vi "ARN Test Konfig.vi"() -> ()   [LabVIEW 2020, in "EPA 1065.lvlib" / "ARN Test 1065-305.lvlib"]
uses:
  ARN Test 1065-305.lvlib
  Allgemein/allgemeine Sub-VIs.lvlib
  Aktion FGV ARN Daten.ctl
  Seiten/FT-IR/FT-IR.lvlib
  Seiten/FT-IR/FGV FT-IR Gasliste Aktionen.ctl
  Messdaten/Aktionen FGV Messdaten.ctl
  Messdaten/Messdaten.lvlib
  Aktion FGV ARN Test.ctl
  Seiten/Grafik/Grafik.lvlib
  Aktion FGV ARN Protokoll.ctl
  Funktionstasten/Funktionstasten.lvlib
  Funktionstasten/Funktionstasten-Aktion.ctl
  Funktionstasten/Zustaende.ctl
  Seiten/Gaszuordnung AO/Gaszuordnung AO.lvlib
  Seiten/Gaszuordnung AO/FGV Gaszuordnung Grenzen&Einheit Aktion.ctl
  Aktion FGV ARN-Protokolleinstellungen.ctl
  Aktion FGV Protokoll.ctl
  ARN Info.ctl
  Visualisierungs Elemente/String - Ausgabefeld.ctl
panel:
  out "E_Rauschen:":sgl format="%#.4g"
  out "E_Wiederholgenauigkeit:":sgl format="%#.4g"
  out "E_Genauigkeit:":sgl format="%#.4g"
  out "Rauschen:":sgl caption="Noise:" format="%#.4g"
  out "Wiederholbarkeit:":sgl format="%#.4g"
  out "Genauigkeit:":sgl caption="Accuracy:" format="%#.4g"
  out "Komponente":T1
  out "Mwert":sgl format="%.3f"
  out "PMwert":sgl format="%.3f"
  out "Wert 1":sgl caption="Konzentration" format="%#.3f"
  out "Graph1":waveform(dbl)(graph)
  in  "Abbrechen":bool caption="Cancel"
  out "Status":string
  out "Tabelle":string[][](table)
  in  "SNR Info":T2 {"Konzentration:" format="%#_5g"; "Gas Aufschaltzeit:" format="%#_5g"}
  in  "Textname:":string
  in  "Pfad:":path=path "D:/IAG_Data/Log" caption="Path:"
  in  "Test Start":bool
  in  "Speichern":bool caption="Save"
  # "ARN Test"
  # "Settings"
  # "Graphic"
  # "Limits:"
  # "Results:"
  # "Accuracy:"
  # "Repeatability:"
  # "Noise:"
  # "±"
  # "x"
  # "Protocol settings"
  # "ARN Test"
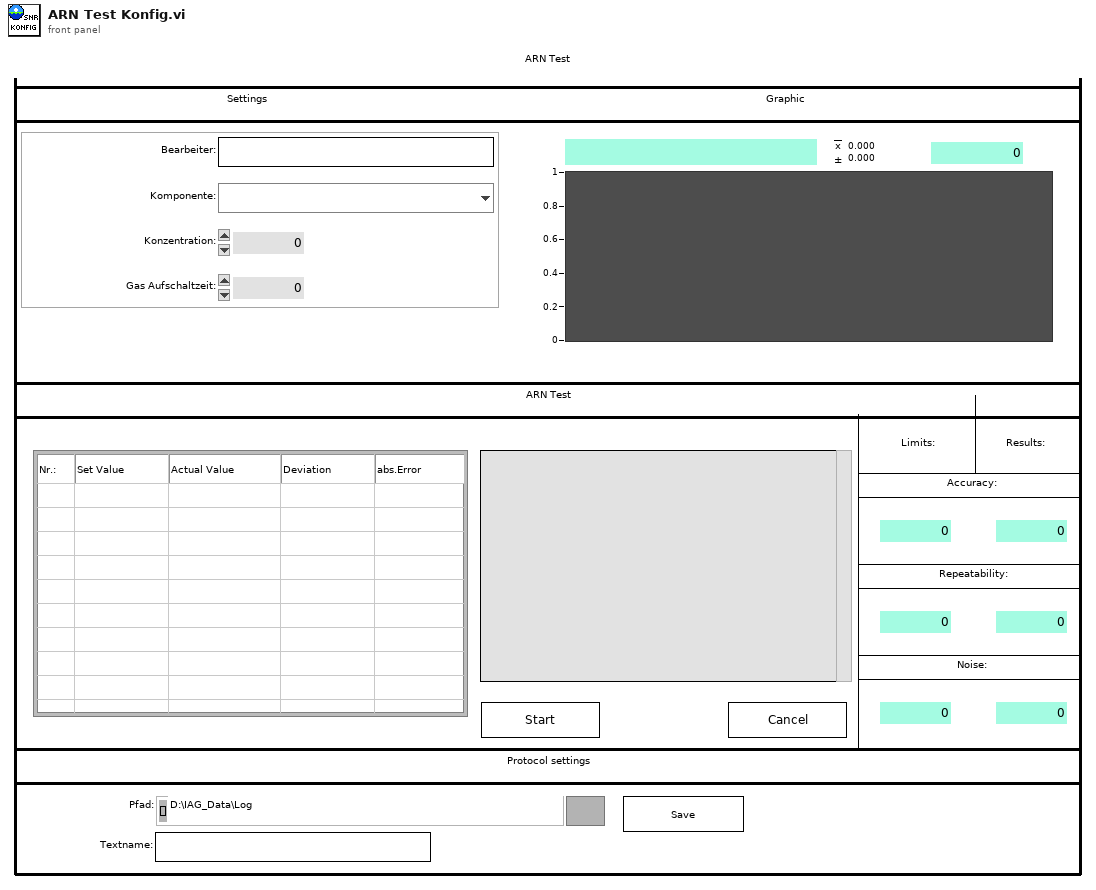
[diagram p1: front panel]
types:
  T1 = typedef "String - Ausgabefeld.ctl" = string
  T2 = typedef "EPA 1065.lvlib/ARN Test 1065-305.lvlib/ARN Info.ctl" = cluster{"Bearbeiter:":string, "Komponente:":u16, "Konzentration:":sgl, "Gas Aufschaltzeit:":sgl}
  T3 = typedef "EPA 1065.lvlib/ARN Test 1065-305.lvlib/Aktion FGV ARN-Protokolleinstellungen.ctl" = enum16{"lesen", "schreiben", "laden", "speichern"}
  T4 = typedef "Messdaten.lvlib/Aktionen FGV Messdaten.ctl" = enum16{"lesen", "schreiben", "löschen", "Mittelwerte", "Komponente"}
  T5 = typedef "EPA 1065.lvlib/ARN Test 1065-305.lvlib/Aktion FGV ARN Test.ctl" = enum16{"leerlauf", "init", "lesen", "CG aufschalten", "Aufschaltzeit abwarten", "aufzeichnen vorbereiten", "aufzeichnen", "berechnen", "auswerten", "fertig", "0-Gas aufschalten", "0-Gas abwarten"}
  T6 = typedef "Gaszuordnung AO.lvlib/FGV Gaszuordnung Grenzen&Einheit Aktion.ctl" = enum16{"Lesen", "Schreiben Min", "Schreiben Max", "Laden", "Speichern"}
  T7 = typedef "EPA 1065.lvlib/ARN Test 1065-305.lvlib/Aktion FGV ARN Protokoll.ctl" = enum16{"lesen", "Tab. schreiben", "Protokoll ausw.", "Protokoll speichern", "Filename", "Pfad"}
  T8 = typedef "FT-IR.lvlib/FGV FT-IR Gasliste Aktionen.ctl" = enum16{"lesen", "Gasliste FT-IR", "Gasliste ausgelesen", "laden", "speichern", "löschen"}
  T9 = typedef "EPA 1065.lvlib/ARN Test 1065-305.lvlib/Aktion FGV ARN Daten.ctl" = enum16{"Lesen", "laden", "speichern", "SNR Info", "Rohdaten", "Rohdaten löschen", "Zeitstempel", "SNR Ergebnis"}
  T10 = typedef "EPA 1065.lvlib/ARN Test 1065-305.lvlib/Allgemeine Einstellungen.ctl" = cluster{"Bearbeiter:":string, "Komponente:":u16, "Gasflaschen Nr.:":string, "Accuracy":dbl, "Sollwert":dbl, "Messgerät:":string, "Seriennummer:":string, "Modus":T11, "Pfad:":path, "Textname:":string, "CG Aufschaltzeit:":dbl, "Einheit":string, "N2 Aufschaltzeit:":dbl}
  T11 = typedef "EPA 1065.lvlib/T90 Test 1065-308.lvlib/Modus.ctl" = u16
  T12 = typedef "EPA 1065.lvlib/ARN Test 1065-305.lvlib/Aktion FGV ARN Protokoll.ctl" = enum16{"lesen", "Tab. schreiben", "Protokoll ausw.", "Protokoll speichern", "Textdatei speichern"}
  T13 = typedef "EPA 1065.lvlib/ARN Test 1065-305.lvlib/Aktion FGV Protokoll.ctl" = enum16{"lesen", "schreiben", "Graph"}
  T14 = typedef "Funktionstasten.lvlib/Zustaende.ctl" = enum16{"Standby", "Pause", "Eco", "Messen", "Kalibrieren", "Spülen Filter", "Spülen Leitung", "Umgebungsluft", "0-Gas", "Cal-Gas", "CG zu PNS", "-------------", "Init 1", "Init 2", "Init 3", "Init 4", "Messen vorbereiten", "Messen durchführen", "Exit"}
  T15 = typedef "Funktionstasten.lvlib/Funktionstasten-Aktion.ctl" = enum16{"Initialisieren", "Zustand setzen", "Taste gedrückt", "Fehler speichern", "Lesen", "Manuell", "Remote", "Bitparallel", "Samplepoint", "Zeit Prüfen", "reset Umschalten"}
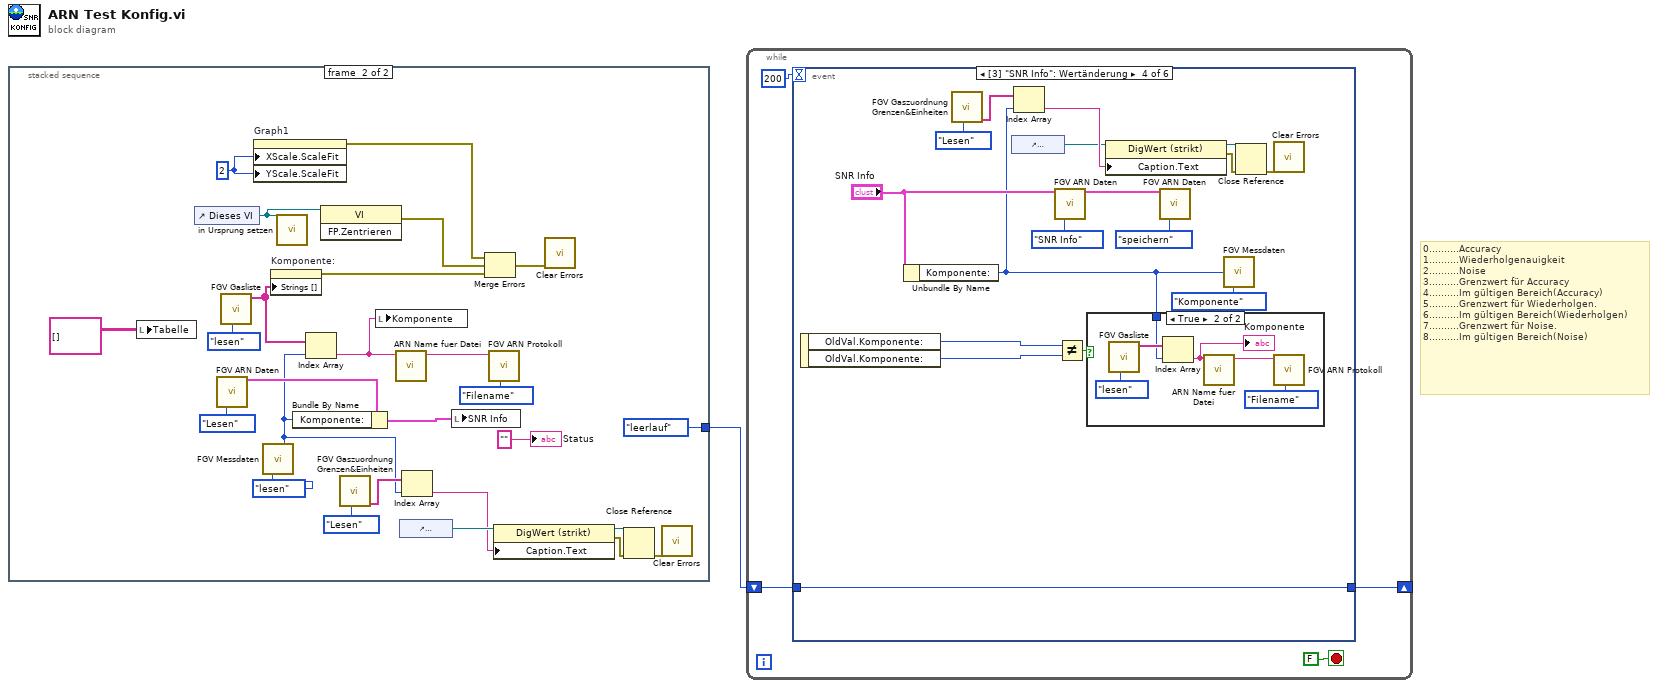
[diagram p0: block diagram]
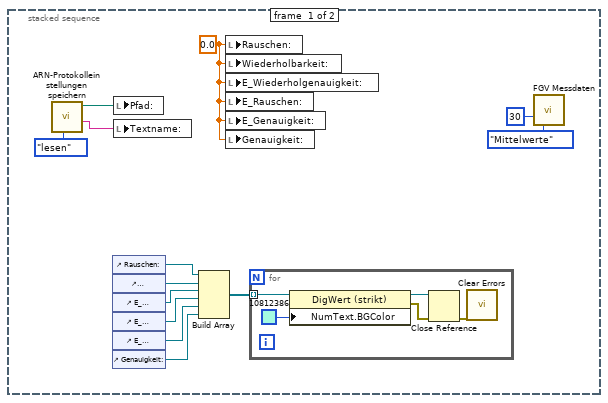
[diagram p2: hidden frame]
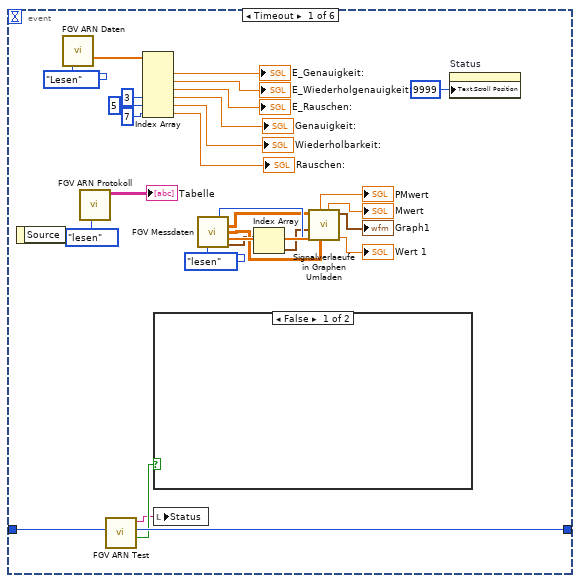
[diagram p3: hidden frame]
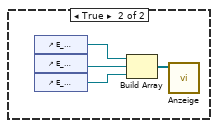
[diagram p4: hidden frame]
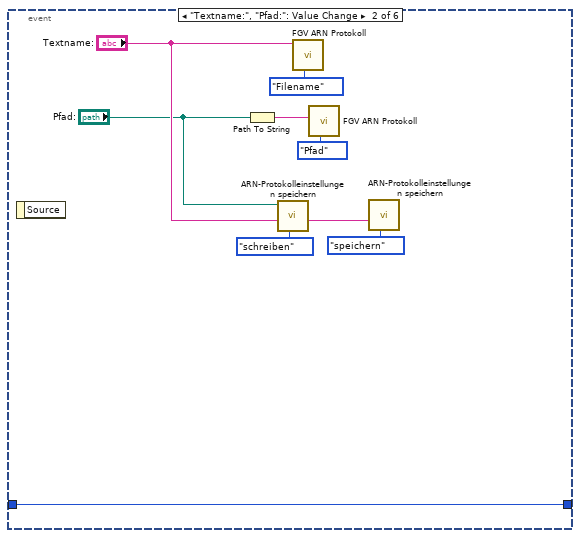
[diagram p5: hidden frame]
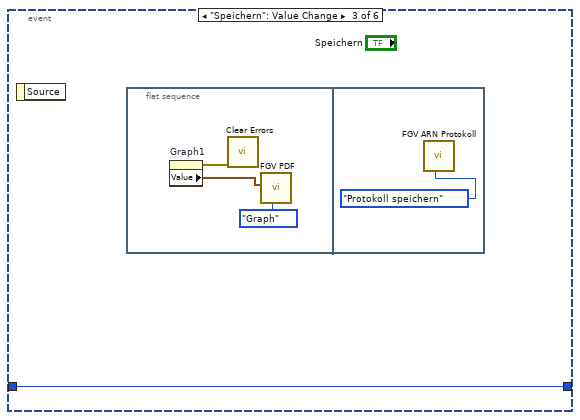
[diagram p6: hidden frame]
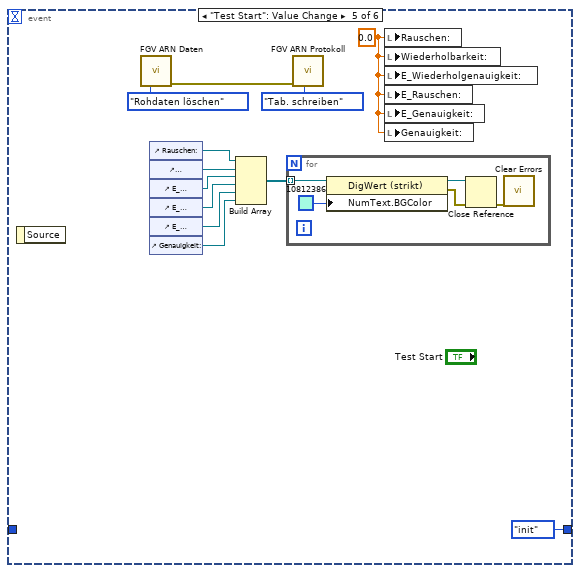
[diagram p8: hidden frame]
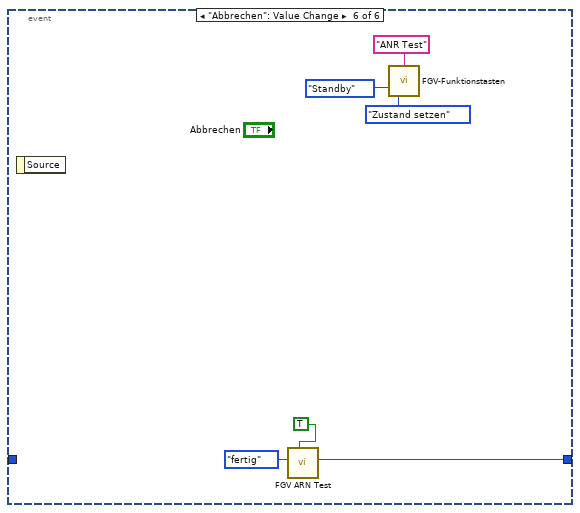
[diagram p9: hidden frame]
diagram:
  # "0..........Accuracy\n1..........Wiederholgenauigkeit\n2..........Noise\n3..........Grenzwert für Accuracy\n4..........Im gültigen Bereich(Accuracy)\n5..........Grenzwert für Wiederholgen.\n6..........Im gültigen Bereich(Wiederholgen)\n7..........Grenzwert für Noise.\n8..........Im gültigen Bereich(Noise)"
  n1 = stacked-sequence {
    tunnel: [_ Aktion_FGV_ARN_Test."leerlauf" ("Aktion")] -> w1
    frame #0 {
      w12 = sgl 0.0 ("Rauschen:")
      n2 = call "ARN-Protokolleinstellungen speichern.vi"("Aktion"=Aktion_FGV_ARN-Protokolleinstellungen."lesen") -> ("Textname"=w2:string, "Pfad"=w3:path)  [unwired: 9 in]
      n3 = control-ref of="Rauschen:"() -> (w11:refnum<vi>)
      n4 = control-ref of="Wiederholbarkeit:"() -> (w10:refnum<vi>)
      n5 = control-ref of="E_Wiederholgenauigkeit:"() -> (w9:refnum<vi>)
      n6 = control-ref of="E_Rauschen:"() -> (w8:refnum<vi>)
      n7 = control-ref of="E_Genauigkeit:"() -> (w7:refnum<vi>)
      n8 = control-ref of="Genauigkeit:"() -> (w6:refnum<vi>)
      n9 = local write "Pfad:"(w3) -> ()
      n10 = local write "Textname:"(w2) -> ()
      n11 = Build Array(w11, w10, w9, w8, w7, w6) -> (w5:refnum<vi>[])
      n12 = local write "Rauschen:"(w12) -> ()
      n13 = local write "Wiederholbarkeit:"(w12) -> ()
      n14 = local write "E_Wiederholgenauigkeit:"(w12) -> ()
      n15 = local write "E_Rauschen:"(w12) -> ()
      n16 = local write "E_Genauigkeit:"(w12) -> ()
      n17 = local write "Genauigkeit:"(w12) -> ()
      n18 = for {
        tunnel: w5 -> [w18] mode=indexing
        n19 = property class="DigWert (strikt)"(reference=w18, "NumText.BGColor"=u32 10812386) -> (reference out=w16:refnum<vi>, error out=w15:errorcluster)  [unwired: 1 in]
        n20 = Close Reference(reference=w16, error in (no error)=w15) -> (error out=w19:errorcluster)
        n21 = call <vilib>:"Clear Errors.vi"("error in (no error)"=w19) -> ()  [unwired: 5 in, 2 out]
      }
      n22 = call "FGV Messdaten.vi"("Mittelwerte"=30, "Aktionen"=Aktionen_FGV_Messdaten."Mittelwerte") -> ()  [unwired: 5 in, 9 out]
    }
    frame #1 {
      w39 = u8 2 ("X-Achse.Achsenanpassung")
      n23 = local write "Tabelle"(string[][] [] ("Tabellenelement")) -> ()
      n24 = control-ref of="Dieses VI"() -> (w31:refnum<vi>)
      n25 = call "FGV ARN Daten.vi"("Aktion"=Aktion_FGV_ARN_Daten."Lesen") -> ("T90 Konfig Daten"=w42:T10)  [unwired: 9 in, 5 out]
      n26 = call "FGV Gasliste.vi"("Aktionen"=FGV_FT-IR_Gasliste_Aktionen."lesen") -> ("Aktuelle Gasliste FT-IR"=w35:T1[])  [unwired: 8 in, 2 out]
      n27 = property on="Graph1" class="SVDiagr (strikt)"("XScale.ScaleFit"=w39, "YScale.ScaleFit"=w39) -> (error out=w38:errorcluster)  [unwired: 2 in, 1 out]
      n28 = call "FGV Messdaten.vi"("Aktionen"=Aktionen_FGV_Messdaten."lesen") -> ("Komponente"=w27:u16)  [unwired: 6 in, 8 out]
      n29 = property on="Komponente:" class="Ring (strikt)"("Strings []"=w35) -> (error out=w37:errorcluster)  [unwired: 2 in, 1 out]
      n30 = call "in Ursprung setzen.vi"("VI Referenz"=w31) -> ()  [unwired: 11 in]
      n31 = Bundle By Name(cluster=w42, "Komponente:"=w27) -> (w41:T10)
      n32 = Index Array(array=w35, index=w27) -> (element=w32:T1)
      n33 = invoke class="VI" method="FP.Zentrieren"(reference=w31) -> (error out=w30:errorcluster)  [unwired: 2 in, 2 out]
      n34 = call "FGV Gaszuordnung Grenzen&Einheiten.vi"("Aktion"=FGV_Gaszuordnung_Grenzen&Einheit_Aktion."Lesen") -> ("Einheit neu"=w28:string[])  [unwired: 2 in, 8 out]
      n35 = local write "Komponente"(w32) -> ()
      n36 = call "ARN Name fuer Datei.vi"("String Eingabe"=w32) -> ("File Name"=w33:string)  [unwired: 10 in]
      n37 = control-ref of="Konzentration:"() -> (w26:refnum<vi>)
      n38 = Index Array(array=w28, index=w27) -> (element=w25:string)
      n39 = local write "SNR Info"(w41) -> ()
      n40 = Merge Errors(w38, w30, w37) -> (w36:errorcluster)
      n41 = call "FGV ARN Protokoll.vi"("Aktion"=Aktion_FGV_ARN_Protokoll."Filename", 11:w33) -> ()  [unwired: 7 in, 3 out]
      n42 = property class="DigWert (strikt)"(reference=w26, "Caption.Text"=w25) -> (reference out=w24:refnum<vi>, error out=w23:errorcluster)  [unwired: 1 in]
      n43 = call <vilib>:"Clear Errors.vi"("error in (no error)"=w36) -> ()  [unwired: 5 in, 2 out]
      n44 = Close Reference(reference=w24, error in (no error)=w23) -> (error out=w22:errorcluster)
      n45 = call <vilib>:"Clear Errors.vi"("error in (no error)"=w22) -> ()  [unwired: 5 in, 2 out]
      "Status" <- "" ("Status")
    }
  }
  n46 = while {
    shift-right: [w46] -> _
    shift-left: w1 -> [w47]
    stop <- FALSE stop-if-true
    n47 = event shown="[3] \"SNR Info\": Wertänderung" {
      selector: _ -> [_ _ _ _ _ _]
      dyn-events: _ -> [_ _ _ _ _ _]
      timeout: 200 -> [_ _ _ _ _ _]
      tunnel: w47 -> [w53 w83 w92 w97 _ _]
      tunnel: [w52 w83 w92 w97 Aktion_FGV_ARN_Test."init" ("Aktion") w137] -> w46
      event Timeout {
        n48 = event-data() -> ()  [unwired: 1 in, 1 out]
        n49 = call "FGV ARN Daten.vi"("Aktion"=Aktion_FGV_ARN_Daten."Lesen") -> ("SNR Ergebnis"=w75:sgl[])  [unwired: 9 in, 5 out]
        n50 = call "FGV ARN Protokoll.vi"("Aktion"=Aktion_FGV_ARN_Protokoll."lesen") -> ("Tabelle"=→"Tabelle":string[][])  [unwired: 8 in, 2 out]
        n51 = call "FGV ARN Test.vi"("Aktion"=w53) -> ("Fertig"=w51:bool, "Aktion"=w52:T5, "Status"=w50:string)  [unwired: 7 in, 1 out]
        n52 = Index Array(array=w75, index #4=3 ("Index"), index #5=5 ("Index"), index #6=7 ("Index")) -> (element #1=→"E_Genauigkeit:":sgl, element #2=→"E_Wiederholgenauigkeit:":sgl, element #3=→"E_Rauschen:":sgl, element #4=→"Genauigkeit:":sgl, element #5=→"Wiederholbarkeit:":sgl, element #6=→"Rauschen:":sgl)  [unwired: 3 in]
        n53 = case shown="False" w51 {
          frame False {
          }
          frame True {
            n54 = control-ref of="E_Genauigkeit:"() -> (w82:refnum<vi>)
            n55 = control-ref of="E_Wiederholgenauigkeit:"() -> (w81:refnum<vi>)
            n56 = control-ref of="E_Rauschen:"() -> (w80:refnum<vi>)
            n57 = Build Array(w82, w81, w80) -> (w79:refnum<vi>[])
            n58 = call "Anzeige.vi"("Anzeigeref."=w79) -> ()  [unwired: 11 in]
          }
        }
        n59 = local write "Status"(w50) -> ()
        n60 = call "FGV Messdaten.vi"("Aktionen"=Aktionen_FGV_Messdaten."lesen") -> ("Komponente"=w62:u16, "Messdaten"=w57:sgl[][], "Mittelwertdaten"=w63:sgl[][], "Deviation"=w64:sgl[], "Zeitstempeln"=w55:timestamp[])  [unwired: 6 in, 4 out]
        n61 = Index Array(array=w55) -> (element=w56:timestamp)  [unwired: 1 in]
        n62 = call "Signalverlaeufe in Graphen Umladen.vi"("Deviation"=w64, "Mittelwertdaten"=w63, "Gas-Auswahl"=w62, "t0"=w56, "Werte"=w57) -> ("Konzentration"=→"Wert 1":sgl, "Waveform"=→"Graph1":waveform(dbl), "aktuelle Mittelwert"=→"Mwert":sgl, "Deviation"=→"PMwert":sgl)  [unwired: 2 in, 1 out]
        n63 = property on="Status" class="Str"("Text.Scroll Position"=u32 9999 ("Text.Anzeigeposition")) -> ()  [unwired: 2 in, 2 out]
      }
      event "Textname:", "Pfad:": Value Change {
        n64 = event-data() -> ()  [unwired: 1 in, 1 out]
        n65 = Path To String(path="Pfad:") -> (string=w89:string)
        n66 = call "ARN-Protokolleinstellungen speichern.vi"("Aktion"=Aktion_FGV_ARN-Protokolleinstellungen."schreiben", "Textname"="Textname:", "Pfad"="Pfad:") -> ("Textname"=w84:string)  [unwired: 7 in, 1 out]
        n67 = call "FGV ARN Protokoll.vi"("Aktion"=Aktion_FGV_ARN_Protokoll."Filename", 11:"Textname:") -> ()  [unwired: 7 in, 3 out]
        n68 = call "FGV ARN Protokoll.vi"("Aktion"=Aktion_FGV_ARN_Protokoll."Pfad", 10:w89) -> ()  [unwired: 7 in, 3 out]
        n69 = call "ARN-Protokolleinstellungen speichern.vi"("Aktion"=Aktion_FGV_ARN-Protokolleinstellungen."speichern", "Textname"=w84) -> ()  [unwired: 8 in, 2 out]
      }
      event "Speichern": Value Change {
        n70 = event-data() -> ()  [unwired: 1 in, 1 out]
        n71 = flat-sequence {
          frame #0 {
            n72 = property on="Graph1" class="SVDiagr (strikt)"() -> (error out=w95:errorcluster, "Value"=w93:waveform(dbl))  [unwired: 2 in, 1 out]
            n73 = call <vilib>:"Clear Errors.vi"("error in (no error)"=w95) -> ()  [unwired: 5 in, 2 out]
            n74 = call "FGV PDF.vi"("Aktion"=Aktion_FGV_Protokoll."Graph", "Graph"=w93) -> ()  [unwired: 8 in, 2 out]
          }
          frame #1 {
            n75 = call "FGV ARN Protokoll.vi"("Aktion"=Aktion_FGV_ARN_Protokoll."Protokoll speichern") -> ()  [unwired: 8 in, 3 out]
          }
        }
      }
      event Value Change {
        n76 = event-data() -> ("OldVal.Komponente:"=w109:u16, "OldVal.Komponente:"=w110:u16)  [unwired: 1 in]
        n77 = Unbundle By Name("SNR Info") -> ("Komponente:"=w105:u16)
        n78 = call "FGV Gaszuordnung Grenzen&Einheiten.vi"("Aktion"=FGV_Gaszuordnung_Grenzen&Einheit_Aktion."Lesen") -> ("Einheit neu"=w99:string[])  [unwired: 2 in, 8 out]
        n79 = control-ref of="Konzentration:"() -> (w100:refnum<vi>)
        n80 = Index Array(array=w99, index=w105) -> (element=w101:string)
        n81 = call "FGV ARN Daten.vi"("T90 Konfig Daten"="SNR Info", "Aktion"=Aktion_FGV_ARN_Daten."SNR Info") -> ("T90 Konfig Daten"=w106:T10)  [unwired: 8 in, 5 out]
        n82 = Not Equal?(x=w109, y=w110) -> (x != y?=w108:bool)
        n83 = case shown="True" w108 {
          tunnel: w105 -> [_ w117]
          frame False {
          }
          frame True {
            n84 = call "FGV Gasliste.vi"("Aktionen"=FGV_FT-IR_Gasliste_Aktionen."lesen") -> ("Aktuelle Gasliste FT-IR"=w119:T1[])  [unwired: 8 in, 2 out]
            n85 = Index Array(array=w119, index=w117) -> (element=w114:T1)
            "Komponente" <- w114
            n86 = call "ARN Name fuer Datei.vi"("String Eingabe"=w114) -> ("File Name"=w115:string)  [unwired: 10 in]
            n87 = call "FGV ARN Protokoll.vi"("Aktion"=Aktion_FGV_ARN_Protokoll."Filename", 11:w115) -> ()  [unwired: 7 in, 3 out]
          }
        }
        n88 = property class="DigWert (strikt)"(reference=w100, "Caption.Text"=w101) -> (reference out=w102:refnum<vi>, error out=w103:errorcluster)  [unwired: 1 in]
        n89 = call "FGV ARN Daten.vi"("T90 Konfig Daten"=w106, "Aktion"=Aktion_FGV_ARN_Daten."speichern") -> ()  [unwired: 8 in, 6 out]
        n90 = call "FGV Messdaten.vi"("Komponente"=w105, "Aktionen"=Aktionen_FGV_Messdaten."Komponente") -> ()  [unwired: 5 in, 9 out]
        n91 = Close Reference(reference=w102, error in (no error)=w103) -> (error out=w104:errorcluster)
        n92 = call <vilib>:"Clear Errors.vi"("error in (no error)"=w104) -> ()  [unwired: 5 in, 2 out]
      }
      event "Test Start": Value Change {
        w131 = sgl 0.0 ("Rauschen:")
        n93 = event-data() -> ()  [unwired: 1 in, 1 out]
        n94 = call "FGV ARN Daten.vi"("Aktion"=Aktion_FGV_ARN_Daten."Rohdaten löschen") -> ("error out"=w121:errorcluster)  [unwired: 9 in, 5 out]
        n95 = control-ref of="Rauschen:"() -> (w124:refnum<vi>)
        n96 = control-ref of="Wiederholbarkeit:"() -> (w125:refnum<vi>)
        n97 = control-ref of="E_Wiederholgenauigkeit:"() -> (w126:refnum<vi>)
        n98 = control-ref of="E_Rauschen:"() -> (w127:refnum<vi>)
        n99 = control-ref of="E_Genauigkeit:"() -> (w128:refnum<vi>)
        n100 = control-ref of="Genauigkeit:"() -> (w129:refnum<vi>)
        n101 = Build Array(w124, w125, w126, w127, w128, w129) -> (w130:refnum<vi>[])
        n102 = for {
          tunnel: w130 -> [w135] mode=indexing
          n103 = property class="DigWert (strikt)"(reference=w135, "NumText.BGColor"=u32 10812386) -> (reference out=w133:refnum<vi>, error out=w132:errorcluster)  [unwired: 1 in]
          n104 = Close Reference(reference=w133, error in (no error)=w132) -> (error out=w136:errorcluster)
          n105 = call <vilib>:"Clear Errors.vi"("error in (no error)"=w136) -> ()  [unwired: 5 in, 2 out]
        }
        n106 = call "FGV ARN Protokoll.vi"("Aktion"=Aktion_FGV_ARN_Protokoll."Tab. schreiben", "error in (no error)"=w121) -> ()  [unwired: 7 in, 3 out]
        n107 = local write "Rauschen:"(w131) -> ()
        n108 = local write "Wiederholbarkeit:"(w131) -> ()
        n109 = local write "E_Wiederholgenauigkeit:"(w131) -> ()
        n110 = local write "E_Rauschen:"(w131) -> ()
        n111 = local write "E_Genauigkeit:"(w131) -> ()
        n112 = local write "Genauigkeit:"(w131) -> ()
      }
      event "Abbrechen": Value Change {
        n113 = event-data() -> ()  [unwired: 1 in, 1 out]
        n114 = call "FGV ARN Test.vi"("abgebrochen"=TRUE, "Aktion"=Aktion_FGV_ARN_Test."fertig") -> ("Aktion"=w137:T5)  [unwired: 6 in, 3 out]
        n115 = call "FGV-Funktionstasten.vi"("Herkunft"="ANR Test", "Zustand"=Zustaende."Standby", "Aktion"=Funktionstasten-Aktion."Zustand setzen") -> ()  [unwired: 7 in, 6 out]
      }
    }
  }
